vi "Begin.vi"(8 "error in":errorcluster) -> (0 "error out":errorcluster)   [LabVIEW 2014]
doc: "Called before other user functions, this VI is expected to open initial I/O refnums, load in file data, and do all program initialization. Notice that the <B>error out</B> terminal is simply used for data flow. Wiring it to other structures or subVIs ensures that this VI runs first."
uses:
  <vilib>/Rock Robotics/WPI/DriverStation/WPI_DriverStationRobotMode2.ctl
  <vilib>/Rock Robotics/WPI/Joystick/WPI_JoystickDeviceEnum.ctl
  <vilib>/Rock Robotics/SystemInterfaces/DIO/FPGA_DIOChannel.ctl
  <vilib>/Rock Robotics/WPI/CAN/TalonSRX/WPI_CANTalonSRX_BrakeOverride.ctl
  <vilib>/Rock Robotics/WPI/Solenoid/WPI_SolenoidChannel.ctl
  <vilib>/Rock Robotics/WPI/Solenoid/WPI_SolenoidValue.ctl
  <vilib>/Rock Robotics/SystemInterfaces/AI/FPGA_AIGyroChannel.ctl
  <vilib>/Rock Robotics/WPI/CAN/TalonSRX/WPI_CANTalonSRX_APIControlMode.ctl
  <vilib>/Rock Robotics/SystemInterfaces/spilib/spi_bus.ctl
  Robot Global Data.vi
  <vilib>/Rock Robotics/WPI/MotorControl/WPI_MotorControlOpenCANTalonSRX.vi
  <vilib>/Rock Robotics/WPI/Switch/WPI_SwitchOpenLimit.vi
  <vilib>/Rock Robotics/WPI/Accelerometer/InternalAccelerometer/WPI_AccelerometerInternalOpen.vi
  <vilib>/Rock Robotics/WPI/Compressor/WPI_CompressorGetSetRefNum.vi
  <vilib>/Rock Robotics/WPI/Solenoid/WPI_SolenoidOpenSingle.vi
  <vilib>/Rock Robotics/WPI/Solenoid/WPI_SolenoidSetEnum.vi
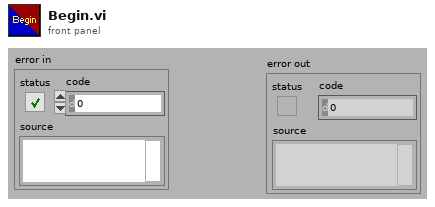
[diagram p1: front panel]
types:
  T1 = typedef "WPI_CANTalonSRX_APIControlMode.ctl" = enum8{"Percent VBus", "Speed", "Position", "Slave", "Unchanged / Invalid"}
  T2 = typedef "FPGA_DIOChannel.ctl" = enum8{"DIO 0", "DIO 1", "DIO 2", "DIO 3", "DIO 4", "DIO 5", "DIO 6", "DIO 7", "DIO 8", "DIO 9", "DIO MXP 0", "DIO MXP 1", "DIO MXP 2", "DIO MXP 3", "DIO MXP 4", "DIO MXP 5", "DIO MXP 6", "DIO MXP 7", "DIO MXP 8", "DIO MXP 9", "DIO MXP 10", "DIO MXP 11", "DIO MXP 12", "DIO MXP 13", "DIO MXP 14", "DIO MXP 15", "Invalid"}
  T3 = typedef "WPI_JoystickDeviceEnum.ctl" = enum16{"USB 0", "USB 1", "USB 2", "USB 3", "USB 4", "USB 5"}
  T4 = typedef "FPGA_AIGyroChannel.ctl" = enum8{"AI 0", "AI 1", "Invalid"}
  T5 = typedef "WPI_SolenoidChannel.ctl" = enum8{"Solenoid 0", "Solenoid 1", "Solenoid 2", "Solenoid 3", "Solenoid 4", "Solenoid 5", "Solenoid 6", "Solenoid 7", "Invalid"}
  T6 = typedef "WPI_SolenoidValue.ctl" = enum16{"Off", "On", "Forward", "Reverse"}
  T7 = typedef "WPI_CANTalonSRX_BrakeOverride.ctl" = enum8{"No Override", "Override to Coast", "Override to Brake"}
  T8 = typedef "WPI_DriverStationRobotMode2.ctl" = enum16{"Autonomous Disabled", "Autonomous Enabled", "Teleop Disabled", "Teleop Enabled", "Disconnected", "Finish", "Test Disabled", "Test Enabled", "Emergency Stopped"}
  T9 = typedef "WPI_MotorControlDeviceRef.ctl" = cluster{"DeviceStatus":errorcluster, "Type":T10, "PWM":cluster{"Controller":T11, "PWM Channel":T12, "DeadBand":T13}, "CAN":cluster{"Device Number":u8, "Control Mode":T14, "Semaphore":T15, "Max Vout":dbl, "TalonSRX Control Mode":T1}, "Invert":bool, "TransformRef":T16, "InvTransformRef":T16}
  T10 = typedef "WPI_MotorControlType.ctl" = enum16{"PWM", "CAN", "CANTalonSRX"}
  T11 = typedef "FPGA_TypedefDigitalModule.ctl" = enum16{"Controller 1"}
  T12 = typedef "FPGA_DIOPWMChannel.ctl" = enum8{"PWM 0", "PWM 1", "PWM 2", "PWM 3", "PWM 4", "PWM 5", "PWM 6", "PWM 7", "PWM 8", "PWM 9", "PWM MXP 0", "PWM MXP 1", "PWM MXP 2", "PWM MXP 3", "PWM MXP 4", "PWM MXP 5", "PWM MXP 6", "PWM MXP 7", "PWM MXP 8", "PWM MXP 9", "Invalid"}
  T13 = typedef "WPI_PWMDeadband.ctl" = cluster{"Name":string, "maxPositivePwm":i32, "minPositivePwm":i32, "centerPwm":i32, "maxNegativePwm":i32, "minNegativePwm":i32, "angularRange":u16}
  T14 = typedef "WPI_CANJaguar_ControlMode.ctl" = enum8{"Percent VBus", "Current", "Speed", "Position", "Voltage"}
  T15 = typedef "Semaphore RefNum" = refnum<k1>
  T16 = typedef "WPI_PWMTransform_ConPane.ctl" = refnum<vi>
  T17 = typedef "WPI_SwitchDevRef.ctl" = cluster{"DevStatus":errorcluster, "DIO Channel":T2, "Controller":T11, "CntIndex":T18, "Normally Closed":bool}
  T18 = typedef "FPGA_CounterCtrSystemIndex.ctl" = enum8{"Ctr 0", "Ctr 1", "Ctr 2", "Ctr 3", "Ctr 4", "Ctr 5", "Ctr 6", "Ctr 7", "Invalid"}
  T19 = typedef "spi_bus.ctl" = enum16{"SPI On-Board, CS0", "SPI On-Board, CS1", "SPI On-Board, CS2", "SPI On-Board, CS3", "SPI MXP", "Invalid"}
  T20 = typedef "WPI_SPIDevRef.ctl" = cluster{"DevStatus":errorcluster, "Handle":i32, "Controller":T11, "SPI Bus":T19}
  T21 = typedef "WPI_AccelerometerDevRef.ctl" = cluster{"DevStatus":errorcluster, "Controller":T22, "Scaling":T23, "Analog Channels":T24, "I2C Bus":T26, "SPI Bus":T19, "Accel Range":T27, "ADXL345 Axes":T28, "Handle":i32, "Device Address":u8, "Accel Type":enum16{"Analog", "ADXL345 I2C", "ADXL345 SPI", "Internal"}}
  T22 = typedef "FPGA_TypedefAnalogModule.ctl" = enum16{"Controller 1"}
  T23 = typedef "WPI_AccelerometerScaling.ctl" = cluster{"Gain (VoltsPerG)":dbl, "Center Voltage":dbl}
  T24 = typedef "WPI_AccelerometerAnalogChannels.ctl" = cluster{"X-Axis":T25, "Y-Axis":T25, "Z-Axis":T25}
  T25 = typedef "FPGA_AIChannel.ctl" = enum8{"AI 0", "AI 1", "AI 2", "AI 3", "AI MXP 0", "AI MXP 1", "AI MXP 2", "AI MXP 3", "Invalid"}
  T26 = typedef "i2c_bus.ctl" = enum16{"I2C On-Board", "I2C MXP", "Invalid"}
  T27 = typedef "ADXL345 Range.ctl" = u8
  T28 = typedef "WPI_AccelerometerADXL345 Axes.ctl" = cluster{"X-Axis":bool, "Y-Axis":bool, "Z-Axis":bool}
  T29 = typedef "WPI_CompressorDevRef.ctl" = cluster{"DevStatus":errorcluster, "Pneumatics Control Module":u8}
  T30 = typedef "WPI_SolenoidDevRef.ctl" = cluster{"DevStatus":errorcluster, "Pneumatics Control Module":u8, "Forward Solenoid Channel":T5, "Reverse Solenoid Channel":T5}
  T31 = typedef "WPI_GyroDevRef.ctl" = cluster{"DevStatus":errorcluster, "Analog Module":T22, "Analog Channel":T25, "Offset":dbl, "Gain (VoltsPerDegree/Second)":dbl}
  T32 = typedef "WPI_JoystickDevRef.ctl" = cluster{"Device":T3}
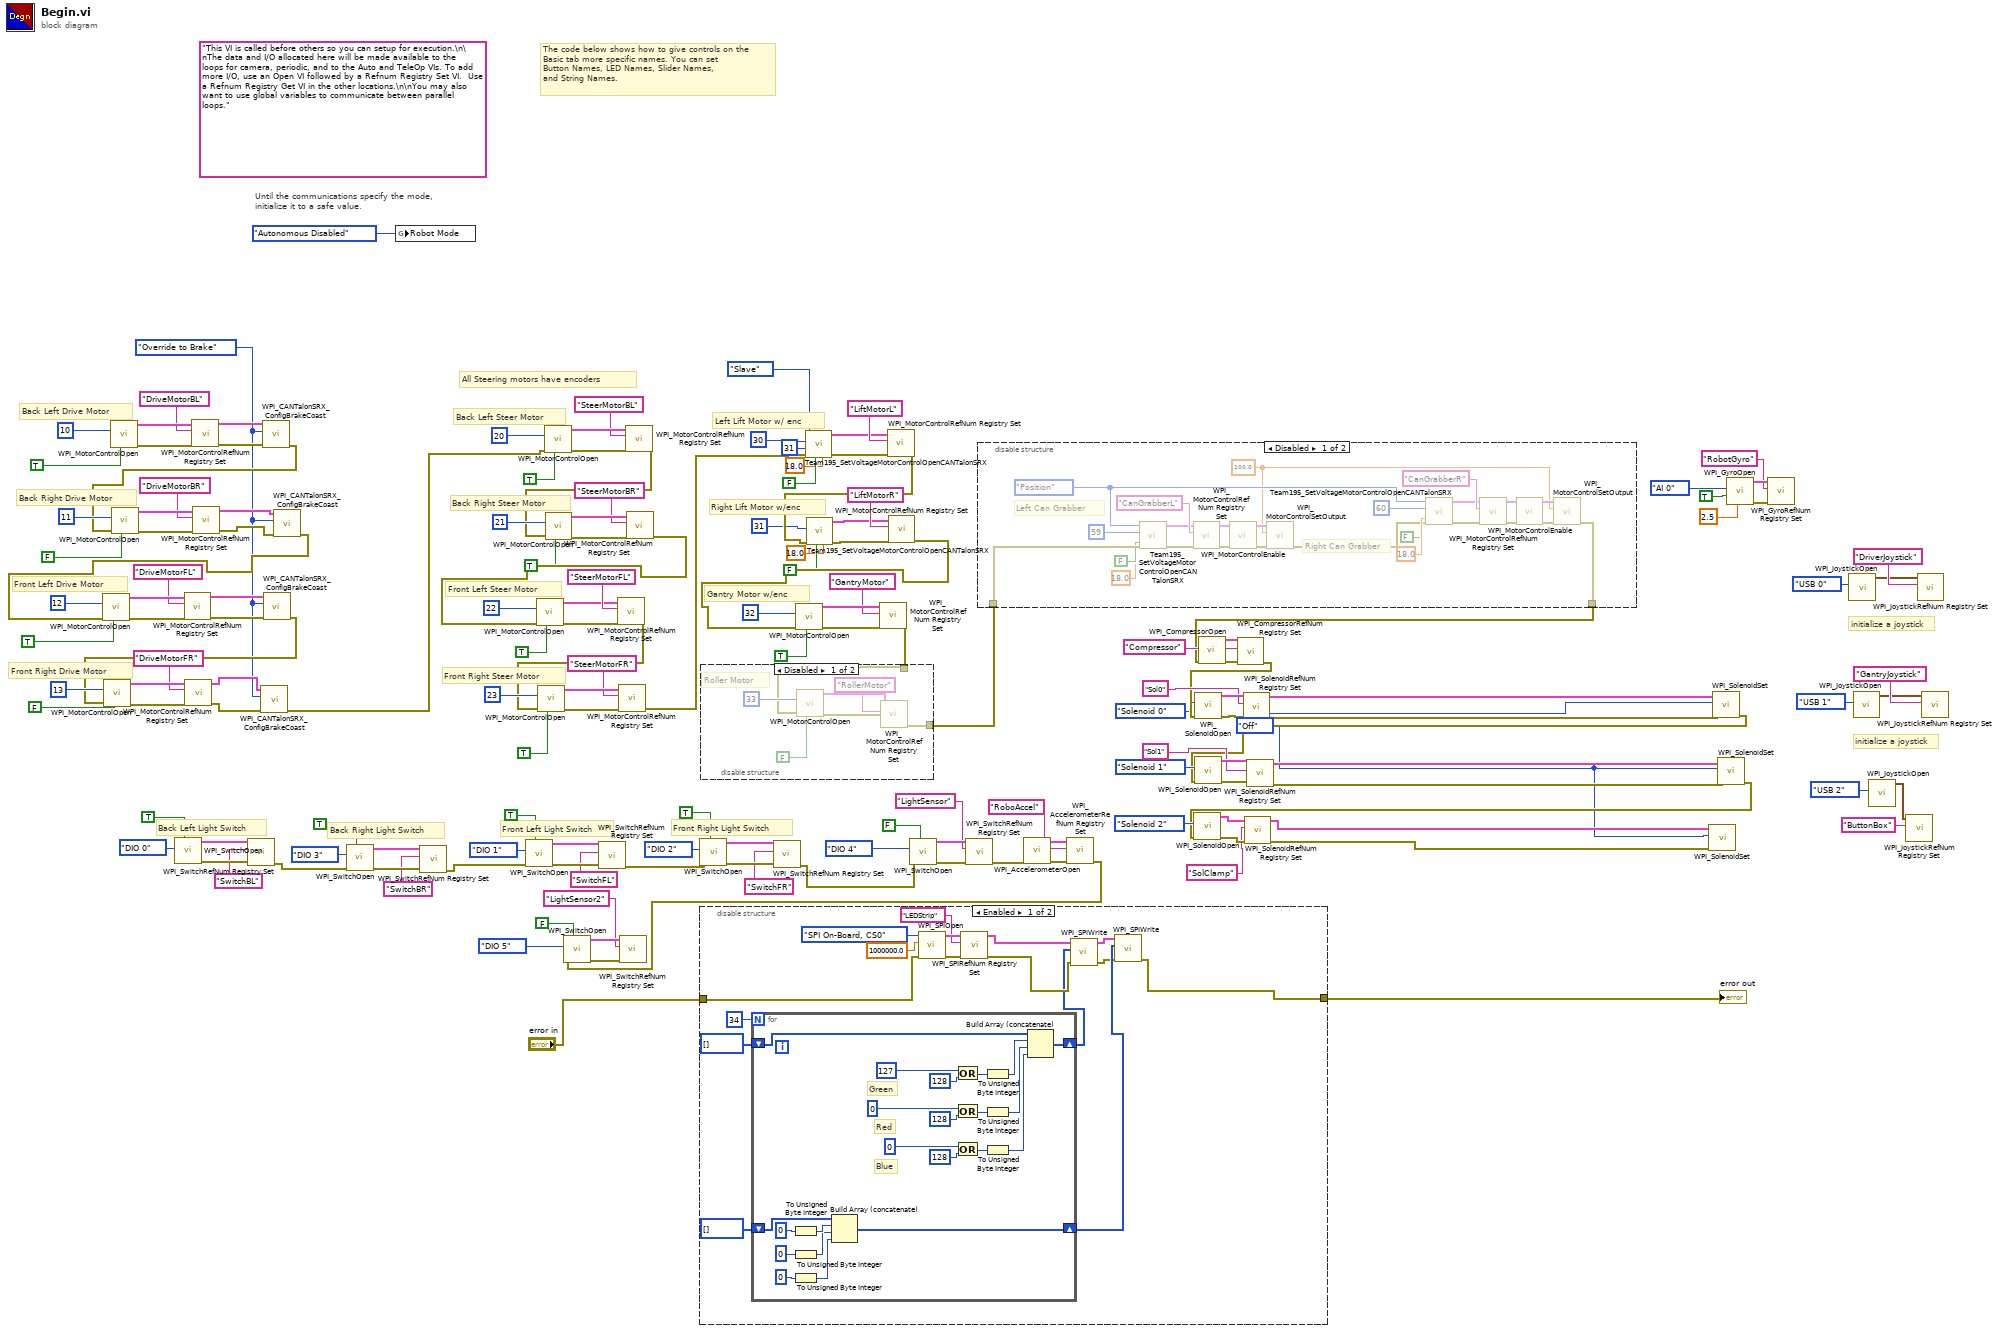
[diagram p0: block diagram]
diagram:
  w29 = WPI_SolenoidValue."Off" ("Value")
  w62 = WPI_CANTalonSRX_BrakeOverride."Override to Brake" ("Brake / Coast Mode")
  (unwired) "This VI is called before others so you can setup for execution.\n\nThe data and I/O allocated here will be made available to the loops for camera, periodic, and to the Auto and TeleOp VIs. To add more I/O, use an Open VI followed by a Refnum Registry Set VI.  Use a Refnum Registry Get VI in the other locations.\n\nYou may also want to use global variables to communicate between parallel loops."
  # "initialize a joystick"
  # "All Steering motors have encoders"
  # "Gantry Motor w/enc"
  # "Right Lift Motor w/enc"
  # "Left Lift Motor w/ enc"
  # "Front Right Light Switch"
  # "Front Left Light Switch"
  # "Back Right Light Switch"
  # "Back Left Light Switch"
  # "Front Right Steer Motor"
  # "Front Left Steer Motor"
  # "Back Right Steer Motor"
  # "Back Left Steer Motor"
  # "Front Right Drive Motor"
  # "Front Left Drive Motor"
  # "Back Right Drive Motor"
  # "Back Left Drive Motor"
  # "The code below shows how to give controls on the\nBasic tab more specific names. You can set\nButton Names, LED Names, Slider Names,\nand String Names."
  # "initialize a joystick"
  # "Until the communications specify the mode,\ninitialize it to a safe value."
  n1 = call-poly <vilib>:"WPI_MotorControlOpen.vi"("Invert"=TRUE, "Device Number"=u8 10) -> ("error out"=w156:errorcluster, "MotorControlDeviceRef"=w158:T9)  [unwired: 8 in]
  n2 = call-poly <vilib>:"WPI_SwitchOpen.vi"("Normally Closed"=TRUE, "DIO Channel"=FPGA_DIOChannel."DIO 0") -> ("error out"=w111:errorcluster, "SwitchDevRef"=w109:T17)  [unwired: 8 in]
  n3 = call <vilib>:"WPI_MotorControlRefNum Registry Set.vi"("error in (no error)"=w156, "refnum name"="DriveMotorBL", "MotorControlDevRef"=w158) -> ("error out"=w74:errorcluster, "MotorControlDevRef"=w72:T9)  [unwired: 7 in]
  n4 = call <vilib>:"WPI_SwitchRefNum Registry Set.vi"("error in (no error)"=w111, "refnum name"="SwitchBL", "SwitchDevRef"=w109) -> ("error out"=w124:errorcluster)  [unwired: 7 in, 1 out]
  n5 = call <vilib>:"WPI_CANTalonSRX_ConfigBrakeCoast.vi"("error in (no error)"=w74, "Brake / Coast Mode"=w62, "CAN Talon SRX Ref"=w72) -> ("error out"=w73:errorcluster)  [unwired: 7 in, 1 out]
  n6 = call-poly <vilib>:"WPI_MotorControlOpen.vi"("Invert"=FALSE, "error in (no error)"=w73, "Device Number"=u8 11) -> ("error out"=w152:errorcluster, "MotorControlDeviceRef"=w154:T9)  [unwired: 7 in]
  n7 = call <vilib>:"WPI_MotorControlRefNum Registry Set.vi"("error in (no error)"=w152, "refnum name"="DriveMotorBR", "MotorControlDevRef"=w154) -> ("error out"=w71:errorcluster, "MotorControlDevRef"=w69:T9)  [unwired: 7 in]
  n8 = call <vilib>:"WPI_CANTalonSRX_ConfigBrakeCoast.vi"("error in (no error)"=w71, "Brake / Coast Mode"=w62, "CAN Talon SRX Ref"=w69) -> ("error out"=w70:errorcluster)  [unwired: 7 in, 1 out]
  n9 = call-poly <vilib>:"WPI_MotorControlOpen.vi"("Invert"=TRUE, "error in (no error)"=w70, "Device Number"=u8 12) -> ("error out"=w148:errorcluster, "MotorControlDeviceRef"=w150:T9)  [unwired: 7 in]
  n10 = call <vilib>:"WPI_MotorControlRefNum Registry Set.vi"("error in (no error)"=w148, "refnum name"="DriveMotorFL", "MotorControlDevRef"=w150) -> ("error out"=w67:errorcluster, "MotorControlDevRef"=w68:T9)  [unwired: 7 in]
  n11 = call <vilib>:"WPI_CANTalonSRX_ConfigBrakeCoast.vi"("error in (no error)"=w67, "Brake / Coast Mode"=w62, "CAN Talon SRX Ref"=w68) -> ("error out"=w66:errorcluster)  [unwired: 7 in, 1 out]
  n12 = call-poly <vilib>:"WPI_MotorControlOpen.vi"("Invert"=FALSE, "error in (no error)"=w66, "Device Number"=u8 13) -> ("error out"=w144:errorcluster, "MotorControlDeviceRef"=w146:T9)  [unwired: 7 in]
  n13 = call <vilib>:"WPI_MotorControlRefNum Registry Set.vi"("error in (no error)"=w144, "refnum name"="DriveMotorFR", "MotorControlDevRef"=w146) -> ("error out"=w65:errorcluster, "MotorControlDevRef"=w64:T9)  [unwired: 7 in]
  n14 = call <vilib>:"WPI_CANTalonSRX_ConfigBrakeCoast.vi"("error in (no error)"=w65, "Brake / Coast Mode"=w62, "CAN Talon SRX Ref"=w64) -> ("error out"=w63:errorcluster)  [unwired: 7 in, 1 out]
  n15 = call-poly <vilib>:"WPI_SwitchOpen.vi"("Normally Closed"=TRUE, "error in (no error)"=w124, "DIO Channel"=FPGA_DIOChannel."DIO 3") -> ("error out"=w115:errorcluster, "SwitchDevRef"=w113:T17)  [unwired: 7 in]
  n16 = global write "Robot Global Data.vi" "Robot Mode"(WPI_DriverStationRobotMode2."Autonomous Disabled" ("Robot Mode")) -> ()
  n17 = call <vilib>:"WPI_SwitchRefNum Registry Set.vi"("error in (no error)"=w115, "refnum name"="SwitchBR", "SwitchDevRef"=w113) -> ("error out"=w125:errorcluster)  [unwired: 7 in, 1 out]
  n18 = call-poly <vilib>:"WPI_SwitchOpen.vi"("Normally Closed"=TRUE, "error in (no error)"=w125, "DIO Channel"=FPGA_DIOChannel."DIO 1") -> ("error out"=w119:errorcluster, "SwitchDevRef"=w117:T17)  [unwired: 7 in]
  n19 = call-poly <vilib>:"WPI_MotorControlOpen.vi"("Invert"=TRUE, "error in (no error)"=w63, "Device Number"=u8 20) -> ("error out"=w140:errorcluster, "MotorControlDeviceRef"=w142:T9)  [unwired: 7 in]
  n20 = call <vilib>:"WPI_SwitchRefNum Registry Set.vi"("error in (no error)"=w119, "refnum name"="SwitchFL", "SwitchDevRef"=w117) -> ("error out"=w126:errorcluster)  [unwired: 7 in, 1 out]
  n21 = call <vilib>:"WPI_MotorControlRefNum Registry Set.vi"("error in (no error)"=w140, "refnum name"="SteerMotorBL", "MotorControlDevRef"=w142) -> ("error out"=w135:errorcluster)  [unwired: 7 in, 1 out]
  n22 = call-poly <vilib>:"WPI_MotorControlOpen.vi"("Invert"=TRUE, "error in (no error)"=w135, "Device Number"=u8 21) -> ("error out"=w136:errorcluster, "MotorControlDeviceRef"=w138:T9)  [unwired: 7 in]
  n23 = call <vilib>:"WPI_MotorControlRefNum Registry Set.vi"("error in (no error)"=w136, "refnum name"="SteerMotorBR", "MotorControlDevRef"=w138) -> ("error out"=w127:errorcluster)  [unwired: 7 in, 1 out]
  n24 = call-poly <vilib>:"WPI_MotorControlOpen.vi"("Invert"=TRUE, "error in (no error)"=w127, "Device Number"=u8 22) -> ("error out"=w40:errorcluster, "MotorControlDeviceRef"=w41:T9)  [unwired: 7 in]
  n25 = call <vilib>:"WPI_MotorControlRefNum Registry Set.vi"("error in (no error)"=w40, "refnum name"="SteerMotorFL", "MotorControlDevRef"=w41) -> ("error out"=w128:errorcluster)  [unwired: 7 in, 1 out]
  n26 = call-poly <vilib>:"WPI_MotorControlOpen.vi"("Invert"=TRUE, "error in (no error)"=w128, "Device Number"=u8 23) -> ("error out"=w129:errorcluster, "MotorControlDeviceRef"=w131:T9)  [unwired: 7 in]
  n27 = call <vilib>:"WPI_MotorControlRefNum Registry Set.vi"("error in (no error)"=w129, "refnum name"="SteerMotorFR", "MotorControlDevRef"=w131) -> ("error out"=w83:errorcluster)  [unwired: 7 in, 1 out]
  n28 = call-poly <vilib>:"WPI_SwitchOpen.vi"("Normally Closed"=TRUE, "error in (no error)"=w126, "DIO Channel"=FPGA_DIOChannel."DIO 2") -> ("error out"=w123:errorcluster, "SwitchDevRef"=w121:T17)  [unwired: 7 in]
  n29 = disable-structure shown="Enabled" {
    disable-tunnel: "error in" -> [w175 w202]
    disable-tunnel: [w173 w202] -> w42
    frame Enabled {
      n30 = for {
        N: 34 -> [_]
        shift-right: [w201] -> w168
        shift-left: u8[] [] -> [w200]
        shift-right: [w190] -> w169
        shift-left: u8[] [] -> [w189]
        # "Blue"
        # "Red"
        # "Green"
        n31 = To Unsigned Byte Integer(number=0) -> (unsigned 8bit integer=w195:u8)
        n32 = To Unsigned Byte Integer(number=0) -> (unsigned 8bit integer=w194:u8)
        n33 = To Unsigned Byte Integer(number=0) -> (unsigned 8bit integer=w193:u8)
        n34 = Build Array (concatenate)(w189, w195, w194, w193) -> (w190:u8[])
        n35 = Or(x=127 ("y"), y=128) -> (x .or. y?=w185:i32)
        n36 = Or(x=0 ("y"), y=128) -> (x .or. y?=w186:i32)
        n37 = Or(x=0 ("y"), y=128) -> (x .or. y?=w187:i32)
        n38 = To Unsigned Byte Integer(number=w185) -> (unsigned 8bit integer=w199:u8)
        n39 = To Unsigned Byte Integer(number=w186) -> (unsigned 8bit integer=w198:u8)
        n40 = To Unsigned Byte Integer(number=w187) -> (unsigned 8bit integer=w197:u8)
        n41 = Build Array (concatenate)(w200, w199, w198, w197) -> (w201:u8[])
      }
      n42 = call <vilib>:"WPI_SPIOpen.vi"("error in"=w175, "Clock Rate (Hz)"=1000000.0, "SPI Bus"=spi_bus."SPI On-Board, CS0") -> ("error out"=w179:errorcluster, "SPIDevRef"=w178:T20)  [unwired: 7 in]
      n43 = call <vilib>:"WPI_SPIRefNum Registry Set.vi"("error in (no error)"=w179, "refnum name"="LEDStrip", "SPIDevRef"=w178) -> ("error out"=w172:errorcluster, "SPIDevRef"=w174:T20)  [unwired: 7 in]
      n44 = call <vilib>:"WPI_SPIWrite.vi"("error in (no error)"=w172, "Data To Send"=w168, "SPIDevRef"=w174) -> ("error out"=w167:errorcluster, "SPIDevRef"=w166:T20)  [unwired: 6 in, 1 out]
      n45 = call <vilib>:"WPI_SPIWrite.vi"("error in (no error)"=w167, "Data To Send"=w169, "SPIDevRef"=w166) -> ("error out"=w173:errorcluster)  [unwired: 6 in, 2 out]
    }
    frame Disabled {
    }
  }
  "error out" <- w42
  n46 = call <vilib>:"WPI_SwitchRefNum Registry Set.vi"("error in (no error)"=w123, "refnum name"="SwitchFR", "SwitchDevRef"=w121) -> ("error out"=w17:errorcluster)  [unwired: 7 in, 1 out]
  n47 = call "Team195_SetVoltageMotorControlOpenCANTalonSRX.vi"("CAN.Max Vout"=18.0, "Invert"=FALSE, "error in (no error)"=w83, "Master Device Number"=u8 31, "Device Number"=u8 30, "Control Mode"=WPI_CANTalonSRX_APIControlMode."Slave") -> ("error out"=w84:errorcluster, "MotorControlDeviceRef"=w85:T9)  [unwired: 4 in]
  n48 = call <vilib>:"WPI_MotorControlRefNum Registry Set.vi"("error in (no error)"=w84, "refnum name"="LiftMotorL", "MotorControlDevRef"=w85) -> ("error out"=w81:errorcluster)  [unwired: 7 in, 1 out]
  n49 = call "Team195_SetVoltageMotorControlOpenCANTalonSRX.vi"("CAN.Max Vout"=18.0, "Invert"=FALSE, "error in (no error)"=w81, "Device Number"=u8 31) -> ("error out"=w78:errorcluster, "MotorControlDeviceRef"=w79:T9)  [unwired: 6 in]
  n50 = call <vilib>:"WPI_MotorControlRefNum Registry Set.vi"("error in (no error)"=w78, "refnum name"="LiftMotorR", "MotorControlDevRef"=w79) -> ("error out"=w91:errorcluster)  [unwired: 7 in, 1 out]
  n51 = call-poly <vilib>:"WPI_MotorControlOpen.vi"("Invert"=TRUE, "error in (no error)"=w91, "Device Number"=u8 32) -> ("error out"=w94:errorcluster, "MotorControlDeviceRef"=w96:T9)  [unwired: 7 in]
  n52 = call <vilib>:"WPI_MotorControlRefNum Registry Set.vi"("error in (no error)"=w94, "refnum name"="GantryMotor", "MotorControlDevRef"=w96) -> ("error out"=w93:errorcluster)  [unwired: 7 in, 1 out]
  n53 = disable-structure shown="Disabled" {
    disable-tunnel: w93 -> [w205 w210]
    disable-tunnel: [w203 w210] -> w75
    frame Disabled {
      # "Roller Motor"
      n54 = call-poly <vilib>:"WPI_MotorControlOpen.vi"("Invert"=FALSE, "error in (no error)"=w205, "Device Number"=u8 33) -> ("error out"=w206:errorcluster, "MotorControlDeviceRef"=w208:T9)  [unwired: 7 in]
      n55 = call <vilib>:"WPI_MotorControlRefNum Registry Set.vi"("error in (no error)"=w206, "refnum name"="RollerMotor", "MotorControlDevRef"=w208) -> ("error out"=w203:errorcluster)  [unwired: 7 in, 1 out]
    }
    frame Enabled {
    }
  }
  n56 = call-poly <vilib>:"WPI_SwitchOpen.vi"("Normally Closed"=FALSE, "error in (no error)"=w17, "DIO Channel"=FPGA_DIOChannel."DIO 4") -> ("error out"=w27:errorcluster, "SwitchDevRef"=w28:T17)  [unwired: 7 in]
  n57 = call <vilib>:"WPI_SwitchRefNum Registry Set.vi"("error in (no error)"=w27, "refnum name"="LightSensor", "SwitchDevRef"=w28) -> ("error out"=w13:errorcluster)  [unwired: 7 in, 1 out]
  n58 = disable-structure shown="Disabled" {
    disable-tunnel: w75 -> [w235 _]
    disable-tunnel: [w234 _] -> w3
    frame Disabled {
      w211 = 100.0 ("Output")
      w217 = WPI_CANTalonSRX_APIControlMode."Position" ("Control Mode")
      # "Right Can Grabber"
      # "Left Can Grabber"
      n59 = call "Team195_SetVoltageMotorControlOpenCANTalonSRX.vi"("CAN.Max Vout"=18.0, "Invert"=FALSE, "error in (no error)"=w235, "Device Number"=u8 59, "Control Mode"=w217) -> ("error out"=w230:errorcluster, "MotorControlDeviceRef"=w231:T9)  [unwired: 5 in]
      n60 = call <vilib>:"WPI_MotorControlRefNum Registry Set.vi"("error in (no error)"=w230, "refnum name"="CanGrabberL", "MotorControlDevRef"=w231) -> ("error out"=w227:errorcluster, "MotorControlDevRef"=w226:T9)  [unwired: 7 in]
      n61 = call <vilib>:"WPI_MotorControlEnable.vi"("error in (no error)"=w227, "CAN Jaguar Ref"=w226) -> ("error out"=w216:errorcluster, "CAN Jaguar Ref Out"=w215:T9)  [unwired: 8 in]
      n62 = call <vilib>:"WPI_MotorControlSetOutput.vi"("error in (no error)"=w216, "Output"=w211, "MotorControlDevRef"=w215) -> ("error out"=w214:errorcluster)  [unwired: 6 in, 2 out]
      n63 = call "Team195_SetVoltageMotorControlOpenCANTalonSRX.vi"("CAN.Max Vout"=18.0, "Invert"=FALSE, "error in (no error)"=w214, "Device Number"=u8 60, "Control Mode"=w217) -> ("error out"=w222:errorcluster, "MotorControlDeviceRef"=w221:T9)  [unwired: 5 in]
      n64 = call <vilib>:"WPI_MotorControlRefNum Registry Set.vi"("error in (no error)"=w222, "refnum name"="CanGrabberR", "MotorControlDevRef"=w221) -> ("error out"=w224:errorcluster, "MotorControlDevRef"=w223:T9)  [unwired: 7 in]
      n65 = call <vilib>:"WPI_MotorControlEnable.vi"("error in (no error)"=w224, "CAN Jaguar Ref"=w223) -> ("error out"=w212:errorcluster, "CAN Jaguar Ref Out"=w213:T9)  [unwired: 8 in]
      n66 = call <vilib>:"WPI_MotorControlSetOutput.vi"("error in (no error)"=w212, "Output"=w211, "MotorControlDevRef"=w213) -> ("error out"=w234:errorcluster)  [unwired: 6 in, 2 out]
    }
    frame Enabled {
    }
  }
  n67 = call-poly <vilib>:"WPI_AccelerometerOpen.vi"("error in"=w13) -> ("error out"=w16:errorcluster, "AccelerometerDevRef"=w15:T21)  [unwired: 9 in]
  n68 = call <vilib>:"WPI_AccelerometerRefNum Registry Set.vi"("error in (no error)"=w16, "refnum name"="RoboAccel", "AccelerometerDevRef"=w15) -> ("error out"=w4:errorcluster)  [unwired: 7 in, 1 out]
  n69 = call-poly <vilib>:"WPI_SwitchOpen.vi"("Normally Closed"=FALSE, "error in (no error)"=w4, "DIO Channel"=FPGA_DIOChannel."DIO 5") -> ("error out"=w8:errorcluster, "SwitchDevRef"=w9:T17)  [unwired: 7 in]
  n70 = call <vilib>:"WPI_SwitchRefNum Registry Set.vi"("error in (no error)"=w8, "refnum name"="LightSensor2", "SwitchDevRef"=w9) -> ()  [unwired: 7 in, 2 out]
  n71 = call <vilib>:"WPI_CompressorOpen.vi"("error in (no error)"=w3) -> ("CompressorDevRef"=w59:T29, "error out"=w60:errorcluster)  [unwired: 13 in]
  n72 = call <vilib>:"WPI_CompressorRefNum Registry Set.vi"("error in (no error)"=w60, "refnum name"="Compressor", "CompressorDevRef"=w59) -> ("error out"=w51:errorcluster)  [unwired: 7 in, 1 out]
  n73 = call-poly <vilib>:"WPI_SolenoidOpen.vi"("error in (no error)"=w51, "Solenoid Channel"=WPI_SolenoidChannel."Solenoid 0") -> ("error out"=w57:errorcluster, "SolenoidDevRef"=w56:T30)  [unwired: 8 in]
  n74 = call <vilib>:"WPI_SolenoidRefNum Registry Set.vi"("error in (no error)"=w57, "refnum name"="Sol0", "SolenoidDevRef"=w56) -> ("error out"=w48:errorcluster, "SolenoidDevRef"=w47:T30)  [unwired: 7 in]
  n75 = call-poly <vilib>:"WPI_SolenoidSet.vi"("error in (no error)"=w48, "Value"=w29, "SolenoidDevRef"=w47) -> ("error out"=w46:errorcluster)  [unwired: 7 in, 1 out]
  n76 = call-poly <vilib>:"WPI_SolenoidOpen.vi"("error in (no error)"=w46, "Solenoid Channel"=WPI_SolenoidChannel."Solenoid 1") -> ("error out"=w54:errorcluster, "SolenoidDevRef"=w55:T30)  [unwired: 8 in]
  n77 = call <vilib>:"WPI_SolenoidRefNum Registry Set.vi"("error in (no error)"=w54, "refnum name"="Sol1", "SolenoidDevRef"=w55) -> ("error out"=w44:errorcluster, "SolenoidDevRef"=w45:T30)  [unwired: 7 in]
  n78 = call-poly <vilib>:"WPI_SolenoidSet.vi"("error in (no error)"=w44, "Value"=w29, "SolenoidDevRef"=w45) -> ("error out"=w32:errorcluster)  [unwired: 7 in, 1 out]
  n79 = call-poly <vilib>:"WPI_SolenoidOpen.vi"("error in (no error)"=w32, "Solenoid Channel"=WPI_SolenoidChannel."Solenoid 2") -> ("error out"=w35:errorcluster, "SolenoidDevRef"=w36:T30)  [unwired: 8 in]
  n80 = call <vilib>:"WPI_SolenoidRefNum Registry Set.vi"("error in (no error)"=w35, "refnum name"="SolClamp", "SolenoidDevRef"=w36) -> ("error out"=w30:errorcluster, "SolenoidDevRef"=w31:T30)  [unwired: 7 in]
  n81 = call-poly <vilib>:"WPI_SolenoidSet.vi"("error in (no error)"=w30, "Value"=w29, "SolenoidDevRef"=w31) -> ()  [unwired: 7 in, 2 out]
  n82 = call <vilib>:"WPI_GyroOpen.vi"("Calibrated Center Voltage"=2.5, "Calibrate On Open"=TRUE, "Analog Channel"=FPGA_AIGyroChannel."AI 0") -> ("error out"=w20:errorcluster, "GyroDevRef"=w19:T31)  [unwired: 6 in, 1 out]
  n83 = call <vilib>:"WPI_GyroRefNum Registry Set.vi"("error in (no error)"=w20, "refnum name"="RobotGyro", "GyroDevRef"=w19) -> ()  [unwired: 7 in, 2 out]
  n84 = call <vilib>:"WPI_JoystickOpen.vi"("JoystickDevice"=WPI_JoystickDeviceEnum."USB 0") -> ("JoystickDevRef"=w161:T32)  [unwired: 10 in]
  n85 = call <vilib>:"WPI_JoystickOpen.vi"("JoystickDevice"=WPI_JoystickDeviceEnum."USB 1") -> ("JoystickDevRef"=w38:T32)  [unwired: 10 in]
  n86 = call <vilib>:"WPI_JoystickOpen.vi"("JoystickDevice"=WPI_JoystickDeviceEnum."USB 2") -> ("JoystickDevRef"=w12:T32)  [unwired: 10 in]
  n87 = call <vilib>:"WPI_JoystickRefNum Registry Set.vi"("refnum name"="ButtonBox", "JoystickDevRef"=w12) -> ()  [unwired: 8 in, 2 out]
  n88 = call <vilib>:"WPI_JoystickRefNum Registry Set.vi"("refnum name"="DriverJoystick", "JoystickDevRef"=w161) -> ()  [unwired: 8 in, 2 out]
  n89 = call <vilib>:"WPI_JoystickRefNum Registry Set.vi"("refnum name"="GantryJoystick", "JoystickDevRef"=w38) -> ()  [unwired: 8 in, 2 out]
